vi "number5-N Queen problem solutions.vi"() -> ()   [LabVIEW 2014]
panel:
  out "Array":bool[][][](array[boolean])
  out "Total Solutions":i32
  # "Use this to check answers ->\n(0~91)"
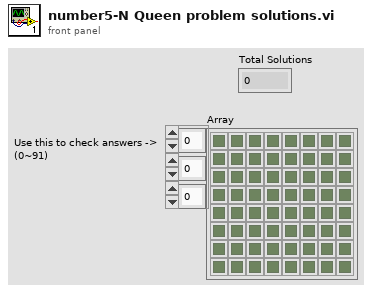
[diagram p1: front panel]
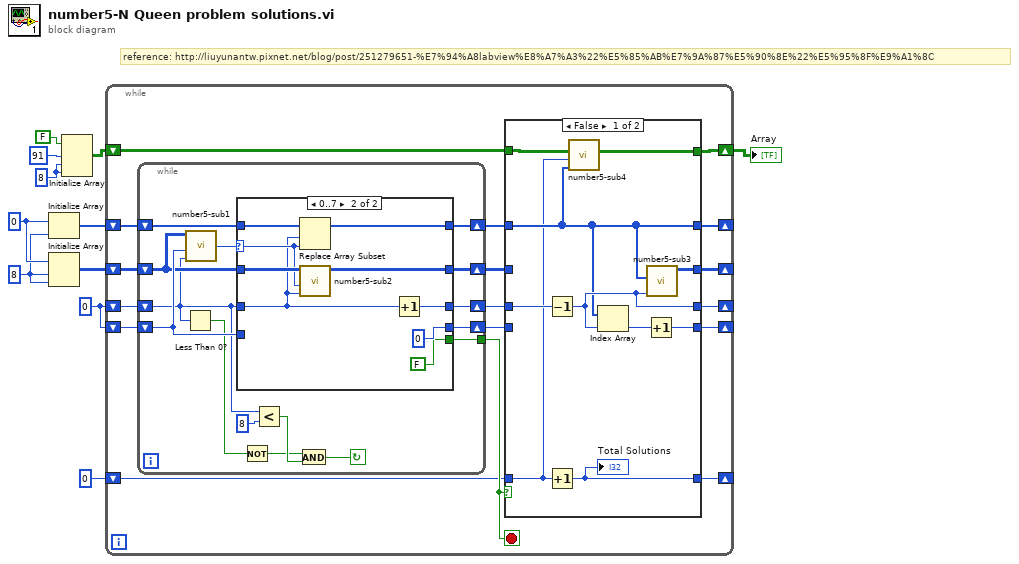
[diagram p0: block diagram]
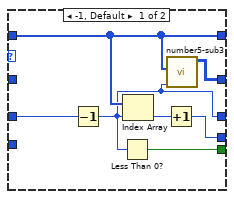
[diagram p3: hidden frame]
diagram:
  w1 = 8 ("dimension size")
  w6 = 0 ("dimension size")
  w8 = 8 ("dimension size")
  w9 = 0 ("dimension size")
  # "reference: http://liuyunantw.pixnet.net/blog/post/251279651-%E7%94%A8labview%E8%A7%A3%22%E5%85%AB%E7%9A%87%E5%90%8E%22%E5%95%8F%E9%A1%8C"
  n1 = Initialize Array(w9, w8) -> (w11:i32[])
  n2 = Initialize Array(w9, w8, w8) -> (w7:i32[][])
  n3 = Initialize Array(FALSE, 91 ("dimension size"), w1, w1) -> (w4:bool[][][])
  n4 = while {
    shift-right: [w17] -> _
    shift-left: w11 -> [w28]
    shift-right: [w18] -> _
    shift-left: 0 ("dimension size") -> [w19]
    shift-right: [w16] -> _
    shift-left: w7 -> [w27]
    shift-right: [w15] -> _
    shift-left: w6 -> [w25]
    shift-right: [w14] -> _
    shift-left: w6 -> [w26]
    shift-right: [w12] -> w3
    shift-left: w4 -> [w13]
    stop <- w20 stop-if-true
    n5 = while {
      shift-right: [w53] -> w21
      shift-left: w25 -> [w49]
      shift-right: [w54] -> w22
      shift-left: w26 -> [w57]
      shift-right: [w46] -> w23
      shift-left: w27 -> [w55]
      shift-right: [w56] -> w24
      shift-left: w28 -> [w59]
      tunnel: [w45] -> w20
      stop <- w52 continue-if-true
      n6 = Less Than 0?(x=w49) -> (x < 0?=w48:bool)
      n7 = call "number5-sub1.vi"("Numeric"=w49, "Numeric 2"=w57, "array"=w55) -> ("index of element"=w58:i32)  [unwired: 3 in]
      n8 = case shown="0..7" w58 {
        selector: w58 -> [_ w71]
        tunnel: w59 -> [w66 w75]
        tunnel: w55 -> [_ w73]
        tunnel: w49 -> [w65 w69]
        tunnel: w57 -> [_ _]
        tunnel: [w66 w74] -> w56
        tunnel: [w60 w72] -> w46
        tunnel: [w62 0 ("dimension size")] -> w54
        tunnel: [w64 w68] -> w53
        tunnel: [w61 FALSE] -> w45
        frame -1, Default {
          n9 = Decrement(x=w65) -> (x-1=w64:i32)
          n10 = Less Than 0?(x=w64) -> (x < 0?=w61:bool)
          n11 = Index Array(array=w66, index=w64) -> (element=w63:i32)
          n12 = Increment(x=w63) -> (x+1=w62:i32)
          n13 = call "number5-sub3.vi"("Numeric"=w64, "Array"=w66) -> ("Array 2"=w60:i32[][])  [unwired: 5 in]
        }
        frame 0..7 {
          n14 = Replace Array Subset(array=w75, new element=w71, index=w69) -> (w74:i32[])
          n15 = call "number5-sub2.vi"("Numeric"=w69, "Numeric 2"=w71, "array"=w73) -> ("array 2"=w72:i32[][])  [unwired: 4 in]
          n16 = Increment(x=w69) -> (x+1=w68:i32)
        }
      }
      n17 = Not(x=w48) -> (.not. x?=w47:bool)
      n18 = Less?(x=w49, y=8 ("dimension size")) -> (x < y?=w51:bool)
      n19 = And(x=w47, y=w51) -> (x .and. y?=w52:bool)
    }
    n20 = case shown="False" w20 {
      tunnel: w24 -> [w31 w43]
      tunnel: w23 -> [_ w42]
      tunnel: w22 -> [_ w41]
      tunnel: w21 -> [w37 w40]
      tunnel: w19 -> [w29 w44]
      tunnel: [w33 w44] -> w18
      tunnel: [w31 w43] -> w17
      tunnel: [w38 w42] -> w16
      tunnel: [w35 w40] -> w15
      tunnel: [w34 w41] -> w14
      tunnel: w13 -> [w30 w39]
      tunnel: [w32 w39] -> w12
      frame False {
        n21 = Decrement(x=w37) -> (x-1=w35:i32)
        n22 = Increment(x=w29) -> (x+1=w33:i32)
        "Total Solutions" <- w33
        n23 = call "number5-sub4.vi"("Array 2"=w31, "index (page)"=w29, "Array 3"=w30) -> ("output array"=w32:bool[][][])  [unwired: 4 in]
        n24 = Index Array(array=w31, index=w35) -> (element=w36:i32)
        n25 = Increment(x=w36) -> (x+1=w34:i32)
        n26 = call "number5-sub3.vi"("Numeric"=w35, "Array"=w31) -> ("Array 2"=w38:i32[][])  [unwired: 5 in]
      }
      frame True {
      }
    }
  }
  "Array" <- w3
